vi "main.vi"() -> ()   [LabVIEW 2024]
uses:
  <vilib>/Utility/error.llb/DialogType.ctl
  <vilib>/DAQmx/read.llb/DAQmx Read (Analog 1D Wfm NChan NSamp).vi
  <vilib>/DAQmx/create/channels.llb/DAQmx Create Channel (AI-Voltage-Basic).vi
  <vilib>/DAQmx/configure/timing.llb/DAQmx Timing (Sample Clock).vi
  <vilib>/DAQmx/configure/task.llb/DAQmx Configure Logging (TDMS).vi
  <vilib>/DAQmx/configure/trigger.llb/DAQmx Start Trigger (Digital Edge).vi
  <vilib>/DAQmx/configure/trigger.llb/DAQmx Start Trigger (Time).vi
  <vilib>/DAQmx/configure/trigger.llb/DAQmx Start Trigger (Analog Edge).vi
  <vilib>/DAQmx/miscellaneous.llb/DAQmx Fill In Error Info.vi
  <vilib>/Utility/file.llb/Read Delimited Spreadsheet (string).vi
  <vilib>/Utility/file.llb/Write Delimited Spreadsheet (string).vi
  <vilib>/Utility/config.llb/Read Key (Double).vi
  <vilib>/Utility/config.llb/Read Key (I32).vi
  <vilib>/Utility/config.llb/Read Key (String).vi
  <vilib>/Utility/config.llb/Read Key (Path).vi
  <vilib>/Utility/config.llb/Write Key (Double).vi
  <vilib>/Utility/config.llb/Write Key (I32).vi
  <vilib>/Utility/config.llb/Write Key (String).vi
  <vilib>/Utility/config.llb/Write Key (Path).vi
  <resource>/objmgr/daqmx.rc
  <vilib>/Utility/config.llb/NI_LVConfig.lvlib
panel:
  in  "?":string(combo)
  out "Waveform Graph 2":waveform(dbl)[](graph)
  in  "?":string(combo)
  out "Waveform Graph":waveform(dbl)[](graph)
  out "子通道数":dbl[](array[numeric])
  in  "配置信息":enum32{"通道信息", "采样信息", "存储信息", "触发信息", "图表显示"}(tab)
  in  "通道信息":i32(listbox)
  in  "Sample Rate":dbl=1000.0
  out "Actual Sample Rate":dbl=1000.0 format="%0.2f"
  in  "Number of Samples":i32=100
  in  "Sample Clock Source":tag="OnboardClock"
  in  "Logging Mode":i32(ring)=10231 items=["Off"=10231, "Log and Read"=15842]
  in  "TDMS File Path":path
  in  "Trigger Type":T1(tab)
  in  "Digital Start Trigger Edge":i32(ring)=10280 caption="Edge" items=["Rising"=10280, "Falling"=10171]
  in  "Digital Start Trigger Source":tag="/Dev1/PFI0" caption="Source"
  in  "Digital Pause Trigger Pause When":i32(ring)=10192 caption="Pause When" items=["High"=10192, "Low"=10214]
  in  "Digital Pause Trigger Source":tag="/Dev1/PFI0" caption="Source"
  in  "Analog Start Trigger Level":dbl caption="Level" format="%0.2f"
  in  "Analog Start Trigger Hysteresis":dbl caption="Hysteresis" format="%.2f"
  in  "Analog Start Trigger Slope":i32(ring)=10280 caption="Slope" items=["Rising"=10280, "Falling"=10171]
  in  "Analog Start Trigger Source":string="APFI0" caption="Source"
  in  "Analog Pause Trigger Source":string="APFI0" caption="Source"
  in  "Analog Pause Trigger Pause When":i32(ring)=10093 caption="Pause When" items=["Above Level"=10093, "Below Level"=10107]
  in  "Analog Pause Trigger Level":dbl caption="Level" format="%.2f"
  in  "When":timestamp
  in  "Select Time\nManually":bool
  in  "横轴（显示时长）":dbl=1000.0
  out "采集状态":bool
  in  "开始采集":bool
  in  "Cluster":T2={"Terminal Configuration"=-1, "Min Voltage"=-5.0, "Physical Channel"="Dev1/ai0", "Max Voltage"=5.0, "function"="", "on/off"=FALSE, "物理量"="", "单位"=""} {"Terminal Configuration" items=["default"=-1, "RSE"=10083, "NRSE"=10078, "Differential"=10106, "Pseudodifferential"=12529]}
  out "Whole Waveform Graph":waveform(dbl)[](graph)
  in  "?":T3(array[cluster]) {"Terminal Configuration" items=["default"=-1, "RSE"=10083, "NRSE"=10078, "Differential"=10106, "Pseudodifferential"=12529]}
  # "All Channels"
  # "Timing Settings"
  # "Logging Settings"
  # "To enable triggers, select a tab above, and configure the settings.\n\nNot all hardware supports all trigger types. Refer to your device documentation for more information."
  # "This trigger type is not supported in continuous sample timing. \n\nRefer to your device documentation for more information on which triggers are supported."
  # "This trigger type is not supported in continuous sample timing. \n\nRefer to your device documentation for more information on which triggers are supported."
  # "If time is not manually set, task will begin after 10 seconds"
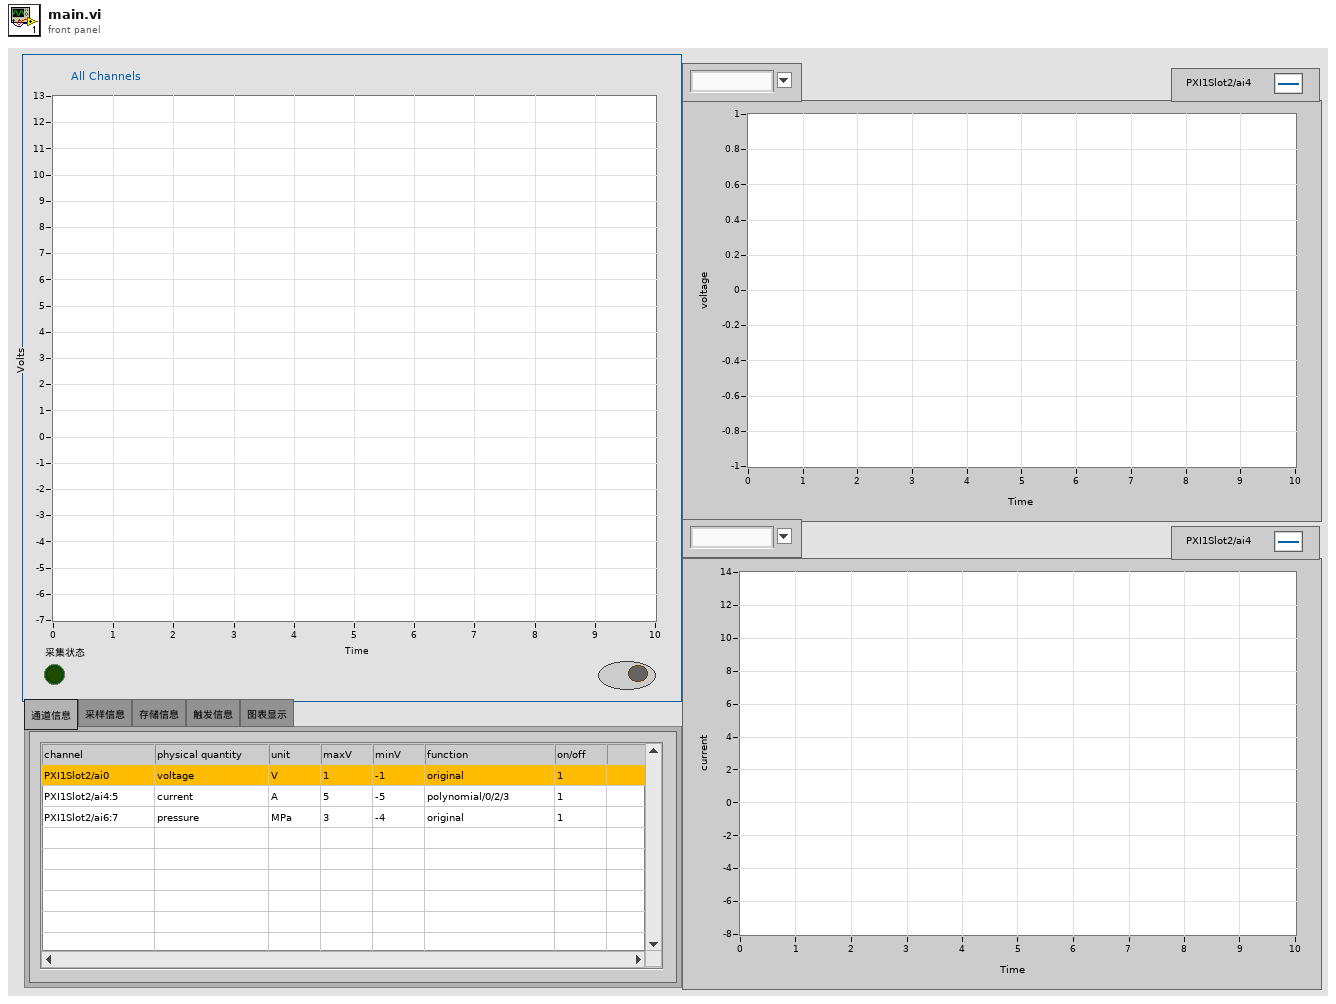
[diagram p1: front panel]
types:
  T1 = enum32{"No Trigger", "Digital Start", "Digital Pause", "Digital Reference", "Analog Start", "Analog Pause", "Analog Reference", "Time Start"}
  T2 = cluster{"Terminal Configuration":i32, "Min Voltage":dbl, "Physical Channel":tag, "Max Voltage":dbl, "function":string, "on/off":bool, "物理量":string, "单位":string}
  T3 = cluster{"Terminal Configuration":i32, "Min Voltage":dbl, "Physical Channel":tag, "Max Voltage":dbl, "function":string, "on/off":bool, "物理量":string, "单位":string}[]
  T4 = typedef "NI_LVConfig.lvlib/Config Data RefNum.ctl" = refnum<k1>
  T5 = typedef "DialogType.ctl" = u16
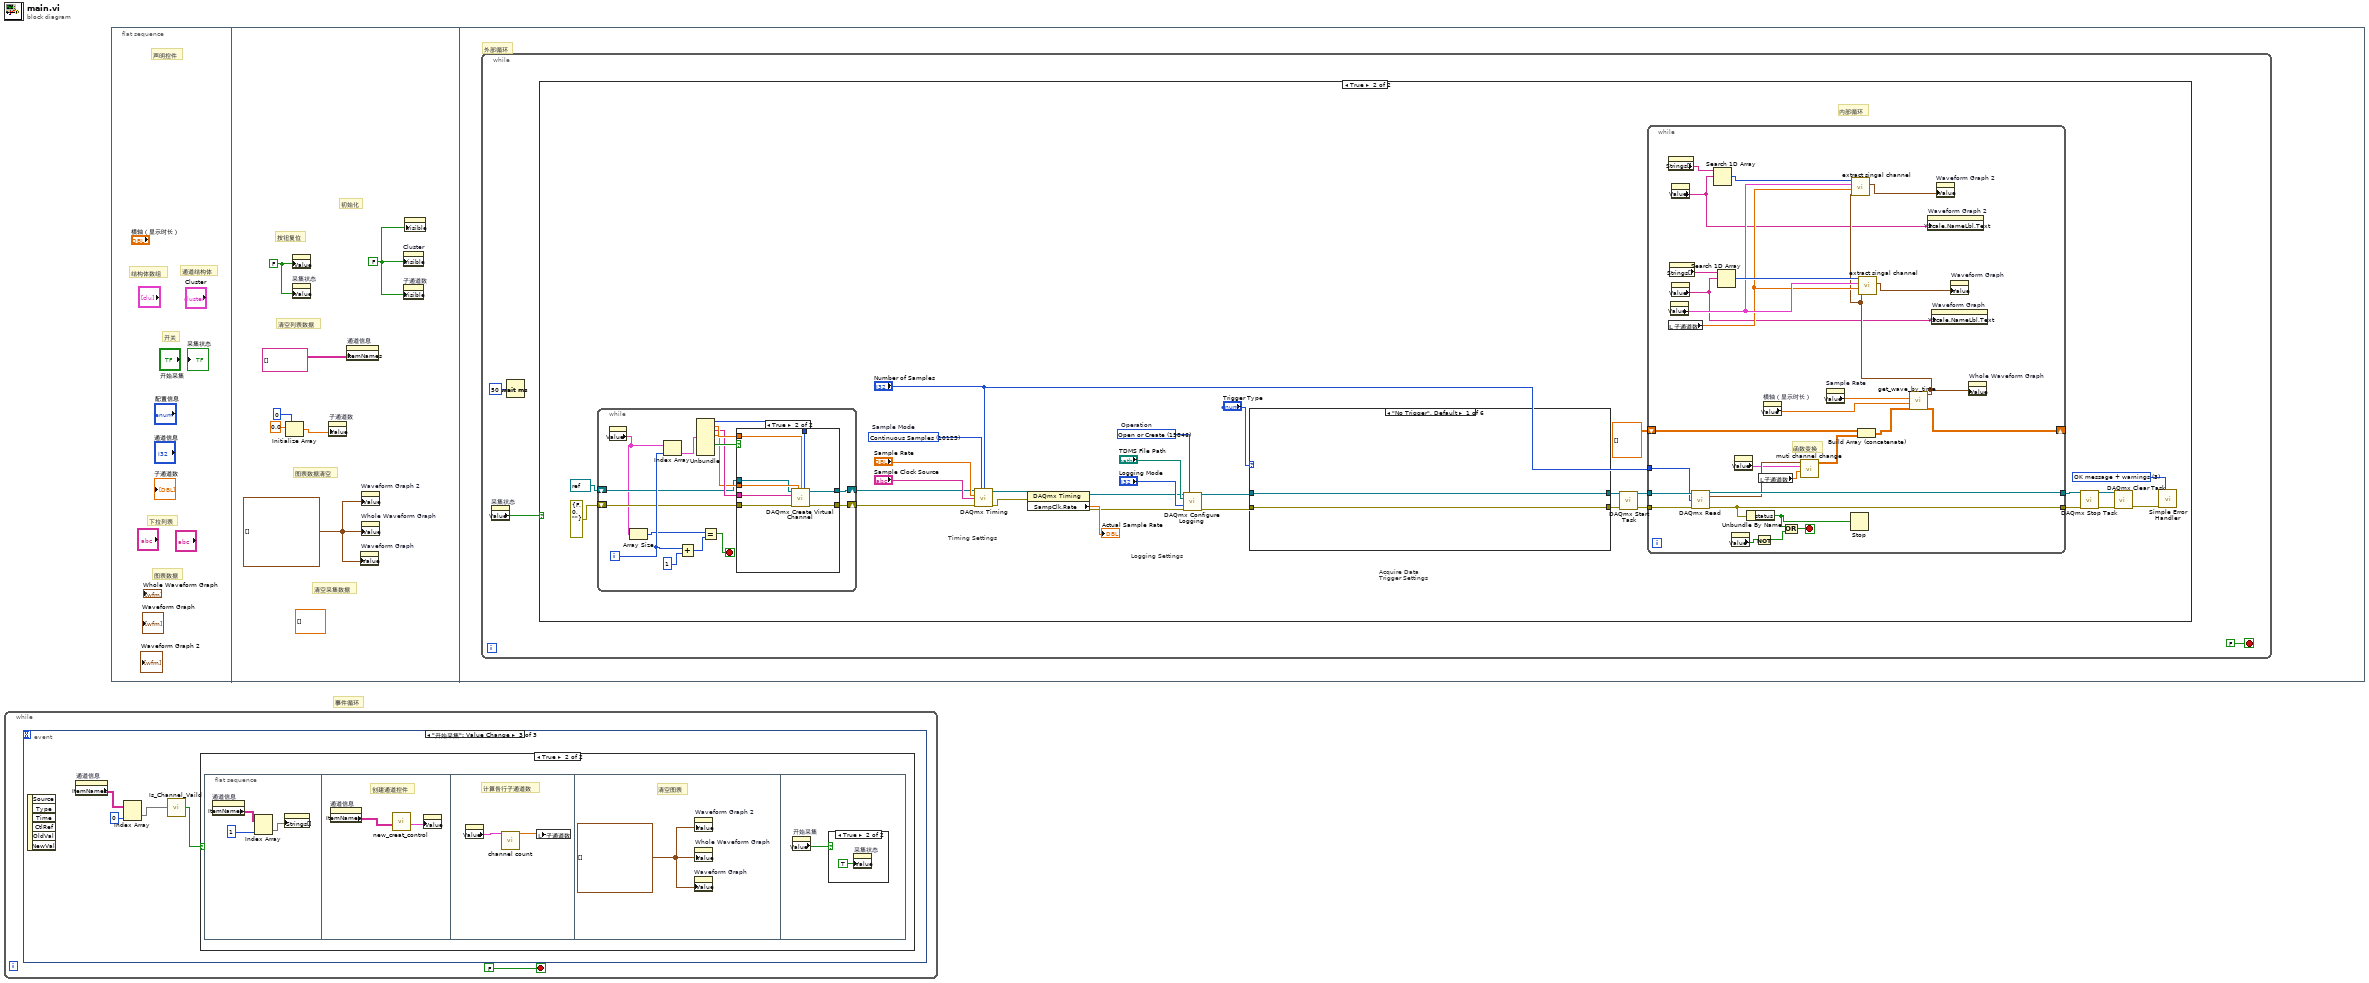
[diagram p0: block diagram]
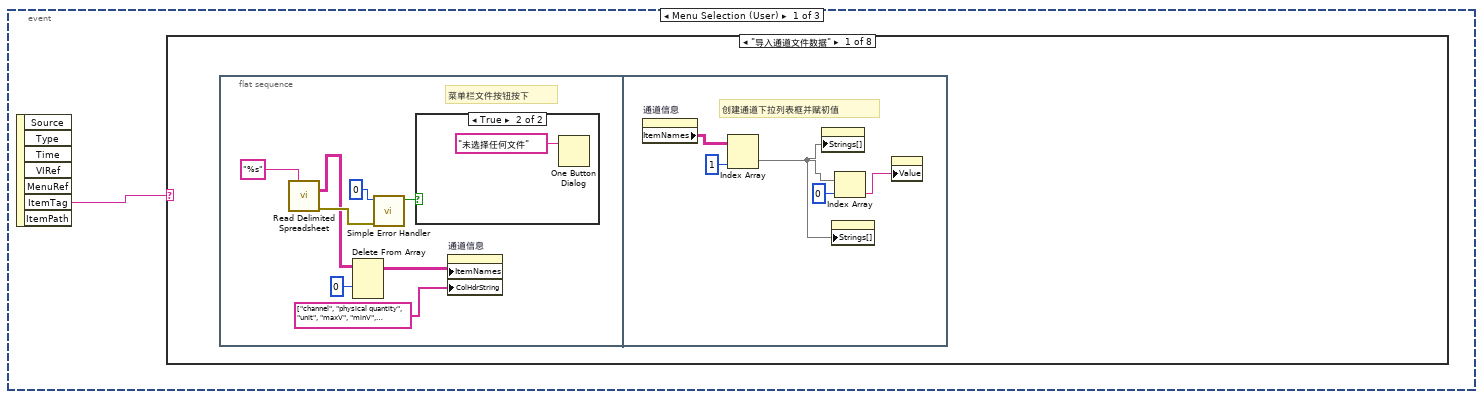
[diagram p2: hidden frame]
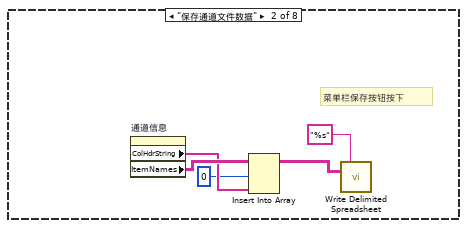
[diagram p4: hidden frame]
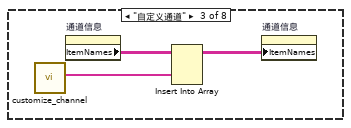
[diagram p5: hidden frame]
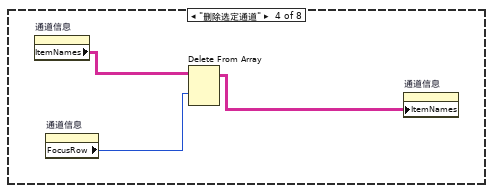
[diagram p6: hidden frame]
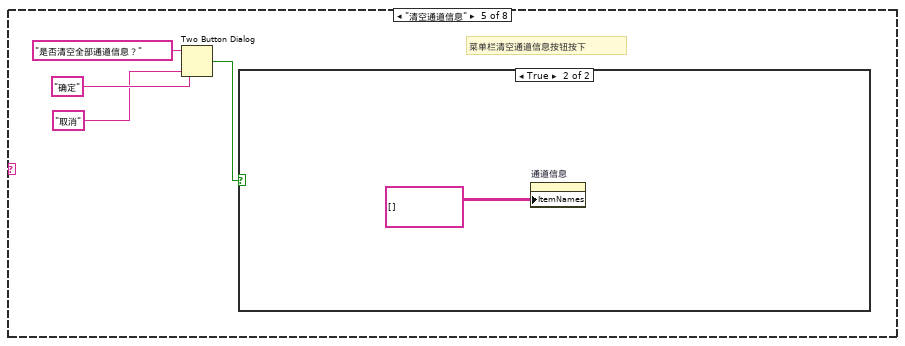
[diagram p7: hidden frame]
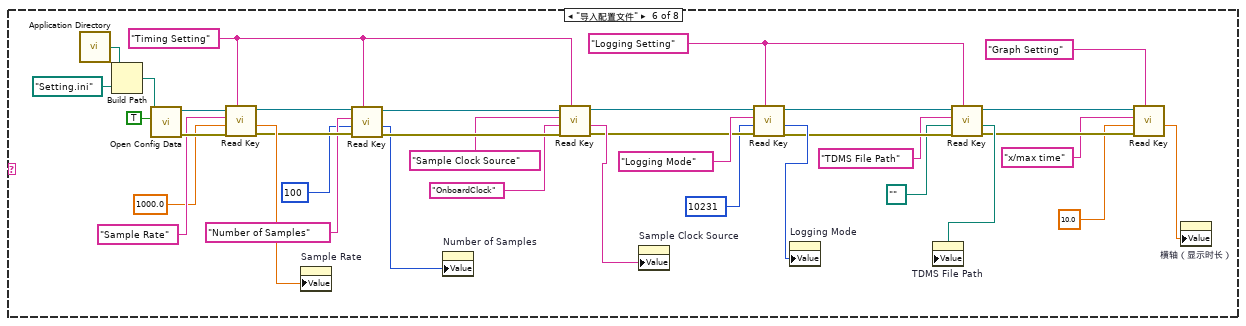
[diagram p9: hidden frame]
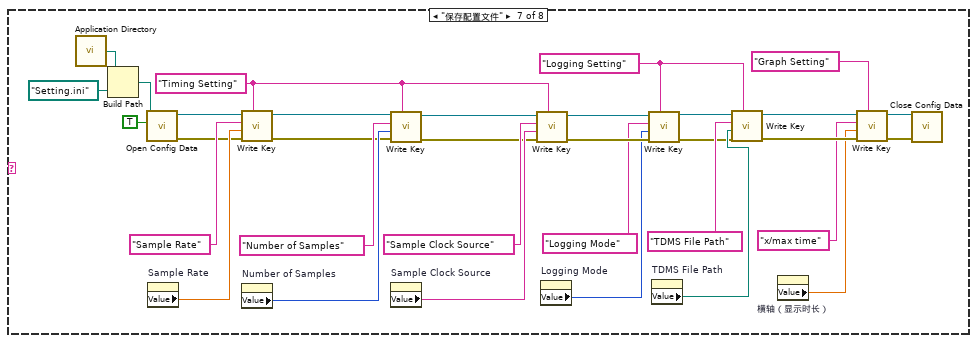
[diagram p10: hidden frame]
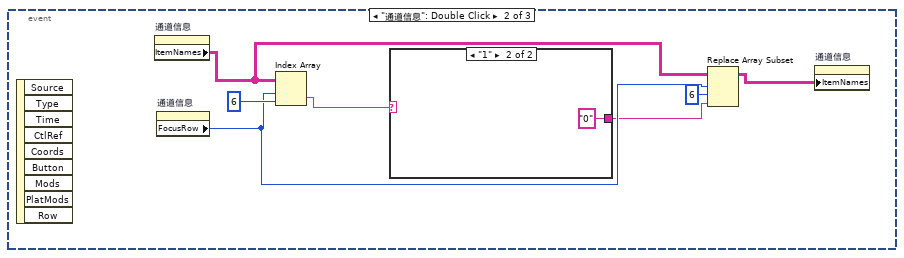
[diagram p12: hidden frame]
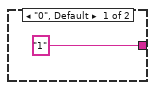
[diagram p13: hidden frame]
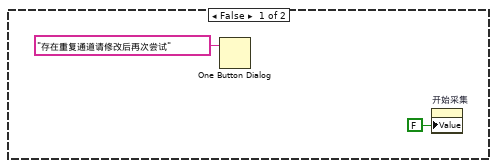
[diagram p14: hidden frame]
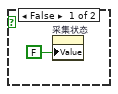
[diagram p15: hidden frame]
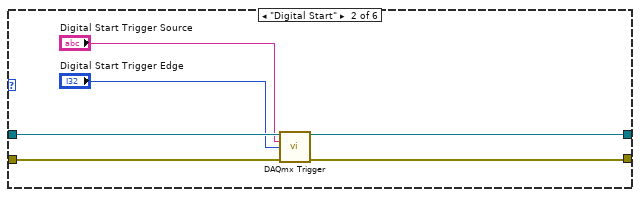
[diagram p17: hidden frame]
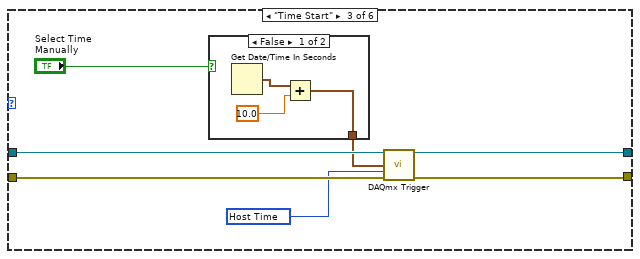
[diagram p18: hidden frame]
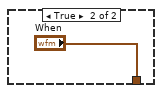
[diagram p19: hidden frame]
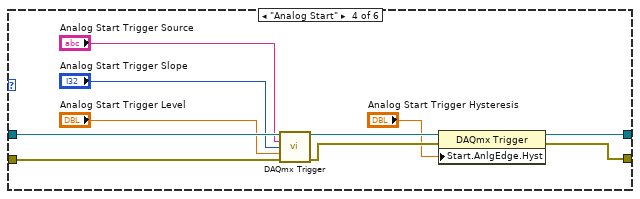
[diagram p20: hidden frame]
diagram:
  # "事件循环"
  n1 = while {
    stop <- FALSE stop-if-true
    n2 = event shown="[2] \"开始采集\": Value Change" {
      selector: _ -> [_ _ _]
      dyn-events: _ -> [_ _ _]
      timeout: _ -> [_ _ _]
      event Menu Selection (User) {
        n3 = event-data() -> ("ItemTag"=w2:string)  [unwired: 1 in, 6 out]
        n4 = case shown="\"导入通道文件数据\"" w2 {
          frame "导入通道文件数据" {
            n5 = flat-sequence {
              frame #0 {
                # "菜单栏文件按钮按下"
                n6 = call-poly <vilib>:"Read Delimited Spreadsheet.vi"("format (%s)"="%s") -> ("all rows"=w8:string[][], "error out"=w10:errorcluster)  [unwired: 9 in, 4 out]
                n7 = Delete From Array(array=w8, index (row)=0) -> (array with subset deleted=w7:string[][])  [unwired: 2 in, 1 out]
                n8 = call <vilib>:"Simple Error Handler.vi"("error code (no error:0)"=0, "error in (no error)"=w10) -> ("error?"=w9:bool)  [unwired: 3 in, 4 out]
                n9 = case shown="True" w9 {
                  frame False {
                  }
                  frame True {
                    n10 = One Button Dialog(message="未选择任何文件") -> ()  [unwired: 1 in, 1 out]
                  }
                }
                n11 = property on="通道信息" class="MCListbox (strict)"("ItemNames"=w7, "ColHdrString"=string[] ["channel", "physical quantity", "unit", "maxV", "minV", "function", "on/off"]) -> ()  [unwired: 2 in, 2 out]
              }
              frame #1 {
                # "创建通道下拉列表框并赋初值"
                n12 = property on="通道信息" class="MCListbox (strict)"() -> ("ItemNames"=w16:string[][])  [unwired: 2 in, 2 out]
                n13 = Index Array(array=w16, index (col)=1 ("disabled index (col)")) -> (element=w12:string[])  [unwired: 1 in]
                n14 = property class="CmbBox"("Strings[]"=w12) -> ()  [unwired: 2 in, 2 out]
                n15 = property class="CmbBox"("Strings[]"=w12) -> ()  [unwired: 2 in, 2 out]
                n16 = Index Array(array=w12, index=0) -> (element=w13:string)
                n17 = property class="CmbBox"("Value"=w13) -> ()  [unwired: 2 in, 2 out]
              }
            }
          }
          frame "保存通道文件数据" {
            # "菜单栏保存按钮按下"
            n18 = property on="通道信息" class="MCListbox (strict)"() -> ("ColHdrString"=w19:string[], "ItemNames"=w20:string[][])  [unwired: 2 in, 2 out]
            n19 = Insert Into Array(array=w20, index (row)=0, new element=w19) -> (w17:string[][])  [unwired: 1 in]
            n20 = call-poly <vilib>:"Write Delimited Spreadsheet.vi"("format (%s)"="%s", "2D data"=w17) -> ()  [unwired: 12 in, 2 out]
          }
          frame "自定义通道" {
            n21 = call "customize_channel.vi"() -> ("Array - String"=w24:string[])  [unwired: 11 in]
            n22 = property on="通道信息" class="MCListbox (strict)"() -> ("ItemNames"=w23:string[][])  [unwired: 2 in, 2 out]
            n23 = Insert Into Array(array=w23, new element=w24) -> (w22:string[][])  [unwired: 2 in]
            n24 = property on="通道信息" class="MCListbox (strict)"("ItemNames"=w22) -> ()  [unwired: 2 in, 2 out]
          }
          frame "删除选定通道" {
            n25 = property on="通道信息" class="MCListbox (strict)"() -> ("ItemNames"=w27:string[][])  [unwired: 2 in, 2 out]
            n26 = property on="通道信息" class="MCListbox (strict)"() -> ("FocusRow"=w26:i32)  [unwired: 2 in, 2 out]
            n27 = Delete From Array(array=w27, index (row)=w26) -> (array with subset deleted=w25:string[][])  [unwired: 2 in, 1 out]
            n28 = property on="通道信息" class="MCListbox (strict)"("ItemNames"=w25) -> ()  [unwired: 2 in, 2 out]
          }
          frame "清空通道信息" {
            # "菜单栏清空通道信息按钮按下"
            n29 = Two Button Dialog(message="是否清空全部通道信息？", 1:"取消" ("F button name (\"Cancel\")"), 2:"确定" ("T button name (\"OK\")")) -> (T button?=w28:bool)
            n30 = case shown="True" w28 {
              frame False {
              }
              frame True {
                n31 = property on="通道信息" class="MCListbox (strict)"("ItemNames"=string[][] []) -> ()  [unwired: 2 in, 2 out]
              }
            }
          }
          frame "导入配置文件" {
            w41 = "Logging Setting" ("section")
            w54 = "Timing Setting" ("section")
            n32 = call <vilib>:"Application Directory.vi"() -> ("Application Directory"=w69:path)
            n33 = Build Path(base path=w69, name or relative path=path "Setting.ini") -> (appended path=w68:path)
            n34 = call <vilib>:"Open Config Data.vi"("create file if necessary (T)"=TRUE, "configuration file path"=w68) -> ("error out"=w64:errorcluster, "refnum"=w65:T4)  [unwired: 7 in, 1 out]
            n35 = call-poly <vilib>:"Read Key.vi"("section"=w54, "error in (no error)"=w64, "default value"=1000.0, "key"="Sample Rate", "refnum"=w65) -> ("error out"=w60:errorcluster, "value"=w62:dbl, "refnum out"=w61:T4)  [unwired: 3 in, 1 out]
            n36 = property on="Sample Rate" class="DigNum (strict)"("Value"=w62) -> ()  [unwired: 2 in, 2 out]
            n37 = call-poly <vilib>:"Read Key.vi"("section"=w54, "error in (no error)"=w60, "default value"=100, "key"="Number of Samples", "refnum"=w61) -> ("error out"=w55:errorcluster, "value"=w53:i32, "refnum out"=w56:T4)  [unwired: 3 in, 1 out]
            n38 = property on="Number of Samples" class="DigNum (strict)"("Value"=w53) -> ()  [unwired: 2 in, 2 out]
            n39 = call-poly <vilib>:"Read Key.vi"("section"=w54, "error in (no error)"=w55, "default value"="OnboardClock", "key"="Sample Clock Source", "refnum"=w56) -> ("error out"=w47:errorcluster, "value"=w50:string, "refnum out"=w48:T4)  [unwired: 3 in, 1 out]
            n40 = property on="Sample Clock Source" class="DAQmxName"("Value"=w50) -> ()  [unwired: 2 in, 2 out]
            n41 = call-poly <vilib>:"Read Key.vi"("section"=w41, "error in (no error)"=w47, "default value"=10231, "key"="Logging Mode", "refnum"=w48) -> ("error out"=w43:errorcluster, "value"=w46:i32, "refnum out"=w44:T4)  [unwired: 3 in, 1 out]
            n42 = property on="Logging Mode" class="Ring (strict)"("Value"=w46) -> ()  [unwired: 2 in, 2 out]
            n43 = call-poly <vilib>:"Read Key.vi"("section"=w41, "error in (no error)"=w43, "default value"=path "", "key"="TDMS File Path", "refnum"=w44) -> ("error out"=w37:errorcluster, "value"=w40:path, "refnum out"=w38:T4)  [unwired: 3 in, 1 out]
            n44 = property on="TDMS File Path" class="Path"("Value"=w40) -> ()  [unwired: 2 in, 2 out]
            n45 = call-poly <vilib>:"Read Key.vi"("section"="Graph Setting", "error in (no error)"=w37, "default value"=10.0, "key"="x/max time", "refnum"=w38) -> ("value"=w34:dbl)  [unwired: 3 in, 3 out]
            n46 = property on="横轴（显示时长）" class="DigNum (strict)"("Value"=w34) -> ()  [unwired: 2 in, 2 out]
          }
          frame "保存配置文件" {
            w81 = "Logging Setting" ("section")
            w92 = "Timing Setting" ("section")
            n47 = call <vilib>:"Application Directory.vi"() -> ("Application Directory"=w88:path)
            n48 = Build Path(base path=w88, name or relative path=path "Setting.ini") -> (appended path=w86:path)
            n49 = call <vilib>:"Open Config Data.vi"("create file if necessary (T)"=TRUE, "configuration file path"=w86) -> ("error out"=w91:errorcluster, "refnum"=w101:T4)  [unwired: 7 in, 1 out]
            n50 = property on="Sample Rate" class="DigNum (strict)"() -> ("Value"=w99:dbl)  [unwired: 2 in, 2 out]
            n51 = call-poly <vilib>:"Write Key.vi"("section"=w92, "error in (no error)"=w91, "value"=w99, "key"="Sample Rate", "refnum"=w101) -> ("error out"=w90:errorcluster, "refnum out"=w98:T4)  [unwired: 4 in, 1 out]
            n52 = property on="Number of Samples" class="DigNum (strict)"() -> ("Value"=w97:i32)  [unwired: 2 in, 2 out]
            n53 = call-poly <vilib>:"Write Key.vi"("section"=w92, "error in (no error)"=w90, "value"=w97, "key"="Number of Samples", "refnum"=w98) -> ("error out"=w89:errorcluster, "refnum out"=w93:T4)  [unwired: 4 in, 1 out]
            n54 = property on="Sample Clock Source" class="DAQmxName"() -> ("Value"=w95:string)  [unwired: 2 in, 2 out]
            n55 = call-poly <vilib>:"Write Key.vi"("section"=w92, "error in (no error)"=w89, "value"=w95, "key"="Sample Clock Source", "refnum"=w93) -> ("error out"=w84:errorcluster, "refnum out"=w85:T4)  [unwired: 4 in, 1 out]
            n56 = property on="Logging Mode" class="Ring (strict)"() -> ("Value"=w83:i32)  [unwired: 2 in, 2 out]
            n57 = call-poly <vilib>:"Write Key.vi"("section"=w81, "error in (no error)"=w84, "value"=w83, "key"="Logging Mode", "refnum"=w85) -> ("error out"=w77:errorcluster, "refnum out"=w78:T4)  [unwired: 4 in, 1 out]
            n58 = property on="TDMS File Path" class="Path"() -> ("Value"=w79:path)  [unwired: 2 in, 2 out]
            n59 = call-poly <vilib>:"Write Key.vi"("section"=w81, "error in (no error)"=w77, "value"=w79, "key"="TDMS File Path", "refnum"=w78) -> ("error out"=w75:errorcluster, "refnum out"=w76:T4)  [unwired: 4 in, 1 out]
            n60 = property on="横轴（显示时长）" class="DigNum (strict)"() -> ("Value"=w73:dbl)  [unwired: 2 in, 2 out]
            n61 = call-poly <vilib>:"Write Key.vi"("section"="Graph Setting", "error in (no error)"=w75, "value"=w73, "key"="x/max time", "refnum"=w76) -> ("error out"=w70:errorcluster, "refnum out"=w71:T4)  [unwired: 4 in, 1 out]
            n62 = call <vilib>:"Close Config Data.vi"("error in (no error)"=w70, "refnum"=w71) -> ()  [unwired: 8 in, 2 out]
          }
          frame "False", Default {
          }
        }
      }
      event "通道信息": Double Click {
        n63 = event-data() -> ()  [unwired: 1 in, 9 out]
        n64 = property on="通道信息" class="MCListbox (strict)"() -> ("ItemNames"=w107:string[][])  [unwired: 2 in, 2 out]
        n65 = property on="通道信息" class="MCListbox (strict)"() -> ("FocusRow"=w105:i32)  [unwired: 2 in, 2 out]
        n66 = Index Array(array=w107, index (row)=w105, index (col)=6 ("disabled index (col)")) -> (element=w108:string)
        n67 = case shown="\"1\"" w108 {
          tunnel: ["1" ("new element/subarray") "0" ("new element/subarray")] -> w104
          frame "0", Default {
          }
          frame "1" {
          }
        }
        n68 = Replace Array Subset(array=w107, new element=w104, index (row)=w105, index (col)=6 ("disabled index (col)")) -> (w103:string[][])
        n69 = property on="通道信息" class="MCListbox (strict)"("ItemNames"=w103) -> ()  [unwired: 2 in, 2 out]
      }
      event "开始采集": Value Change {
        n70 = event-data() -> ()  [unwired: 1 in, 6 out]
        n71 = property on="通道信息" class="MCListbox (strict)"() -> ("ItemNames"=w114:string[][])  [unwired: 2 in, 2 out]
        n72 = Index Array(array=w114, index (col)=0 ("disabled index (col)")) -> (element=w115:string[])  [unwired: 1 in]
        n73 = call "Is_Channel_Vaild.vi"("输入数组"=w115) -> ("元素不重复？（真：不重复，假：有重复元素）"=w112:bool)
        n74 = case shown="True" w112 {
          frame False {
            n75 = One Button Dialog(message="存在重复通道请修改后再次尝试") -> ()  [unwired: 1 in, 1 out]
            n76 = property on="开始采集" class="Bool (strict)"("Value"=FALSE ("开始采集")) -> ()  [unwired: 2 in, 2 out]
          }
          frame True {
            n77 = flat-sequence {
              frame #0 {
                n78 = property on="通道信息" class="MCListbox (strict)"() -> ("ItemNames"=w119:string[][])  [unwired: 2 in, 2 out]
                n79 = Index Array(array=w119, index (col)=1) -> (element=w118:string[])  [unwired: 1 in]
                n80 = property class="CmbBox"("Strings[]"=w118) -> ()  [unwired: 2 in, 2 out]
              }
              frame #1 {
                # "创建通道控件"
                n81 = property on="通道信息" class="MCListbox (strict)"() -> ("ItemNames"=w121:string[][])  [unwired: 2 in, 2 out]
                n82 = call "new_creat_control.vi"("Table"=w121) -> ("Array"=w122:T3)  [unwired: 10 in]
                n83 = property class="Arr (strict)"("Value"=w122) -> ()  [unwired: 2 in, 2 out]
              }
              frame #2 {
                # "计算各行子通道数"
                n84 = property class="Arr (strict)"() -> ("Value"=w124:T3)  [unwired: 2 in, 2 out]
                n85 = call "channel count.vi"(11:w124) -> ("Array - Numeric"=w123:dbl[])  [unwired: 10 in]
                n86 = local write "子通道数"(w123) -> ()
              }
              frame #3 {
                w125 = waveform(dbl)[] [] ("Whole Waveform Graph")
                # "清空图表"
                n87 = property on="Waveform Graph" class="WFGraph (strict)"("Value"=w125) -> ()  [unwired: 2 in, 2 out]
                n88 = property on="Waveform Graph 2" class="WFGraph (strict)"("Value"=w125) -> ()  [unwired: 2 in, 2 out]
                n89 = property on="Whole Waveform Graph" class="WFGraph (strict)"("Value"=w125) -> ()  [unwired: 2 in, 2 out]
              }
              frame #4 {
                n90 = property on="开始采集" class="Bool (strict)"() -> ("Value"=w126:bool)  [unwired: 2 in, 2 out]
                n91 = case shown="True" w126 {
                  frame False {
                    n92 = property on="采集状态" class="Bool (strict)"("Value"=FALSE) -> ()  [unwired: 2 in, 2 out]
                  }
                  frame True {
                    n93 = property on="采集状态" class="Bool (strict)"("Value"=TRUE) -> ()  [unwired: 2 in, 2 out]
                  }
                }
              }
            }
          }
        }
      }
    }
  }
  n94 = flat-sequence {
    frame #0 {
      # "图表数据"
      # "下拉列表"
      # "声明控件"
      # "开关"
      # "结构体数组"
      # "通道结构体"
    }
    frame #1 {
      (unwired) dbl[][] [] ("statistic")
      w129 = waveform(dbl)[] [] ("Whole Waveform Graph")
      w130 = FALSE
      w135 = FALSE ("on/off")
      # "清空采集数据"
      # "图表数据清空"
      # "清空列表数据"
      # "初始化"
      # "按钮复位"
      n95 = Initialize Array(0.0 ("element"), 0 ("dimension size")) -> (w133:dbl[])
      n96 = property on="开始采集" class="Bool (strict)"("Value"=w135) -> ()  [unwired: 2 in, 2 out]
      n97 = property on="采集状态" class="Bool (strict)"("Value"=w135) -> ()  [unwired: 2 in, 2 out]
      n98 = property on="子通道数" class="Arr (strict)"("Value"=w133) -> ()  [unwired: 2 in, 2 out]
      n99 = property on="通道信息" class="MCListbox (strict)"("ItemNames"=string[][] []) -> ()  [unwired: 2 in, 2 out]
      n100 = property on="Waveform Graph" class="WFGraph (strict)"("Value"=w129) -> ()  [unwired: 2 in, 2 out]
      n101 = property on="Waveform Graph 2" class="WFGraph (strict)"("Value"=w129) -> ()  [unwired: 2 in, 2 out]
      n102 = property on="Whole Waveform Graph" class="WFGraph (strict)"("Value"=w129) -> ()  [unwired: 2 in, 2 out]
      n103 = property on="Cluster" class="Clust (strict)"("Visible"=w130) -> ()  [unwired: 2 in, 2 out]
      n104 = property on="子通道数" class="Arr (strict)"("Visible"=w130) -> ()  [unwired: 2 in, 2 out]
      n105 = property class="Arr (strict)"("Visible"=w130) -> ()  [unwired: 2 in, 2 out]
    }
    frame #2 {
      # "外部循环"
      n106 = while {
        stop <- FALSE stop-if-true
        n107 = property on="采集状态" class="Bool (strict)"() -> ("Value"=w136:bool)  [unwired: 2 in, 2 out]
        n108 = Wait (ms)(milliseconds to wait=u32 50) -> ()  [unwired: 1 out]
        n109 = case shown="True" w136 {
          frame False {
          }
          frame True {
            w161 = T5 3 items=["no dialog", "OK message", "continue or stop message", "OK message + warnings", "continue/stop + warnings"] ("type of dialog (OK msg:1)")
            w147 = 15846 items=["Open"=10437, "Open or Create"=15846, "Create or Replace"=15847, "Create"=15848]  # Operation
            w144 = 10123 items=["Finite Samples"=10178, "Continuous Samples"=10123, "Hardware Timed Single Point"=12522]  # Sample Mode
            # "内部循环"
            # "Trigger Settings"
            # "Acquire Data"
            # "Timing Settings"
            # "Logging Settings"
            n110 = while {
              shift-right: [w246] -> w141
              shift-left: refnum<k21> refnum ("task out") -> [w243]
              shift-right: [w245] -> w140
              shift-left: errorcluster {"status"=FALSE, "code"=0, "source"=""} ("error out") -> [w244]
              i -> [w257]
              stop <- w254 stop-if-true
              n111 = property class="Arr (strict)"() -> ("Value"=w242:T3)  [unwired: 2 in, 2 out]
              n112 = Array Size(array=w242) -> (size(s)=w251:i32)
              n113 = Index Array(array=w242, index=w257) -> (element=w253:T2)
              n114 = Add(x=w257, y=1) -> (x+y=w255:i32)
              n115 = Unbundle(w253) -> ("Terminal Configuration"=w250:i32, "Min Voltage"=w249:dbl, "Physical Channel"=w248:tag, "Max Voltage"=w247:dbl, "on/off"=w252:bool)  [unwired: 3 out]
              n116 = Equal?(x=w251, y=w255) -> (x = y?=w254:bool)
              n117 = case shown="True" w252 {
                tunnel: w250 -> [_ w267]
                tunnel: w249 -> [_ w266]
                tunnel: w248 -> [_ w265]
                tunnel: w247 -> [_ w264]
                tunnel: [w259 w263] -> w246
                tunnel: [w258 w262] -> w245
                tunnel: w244 -> [w258 w261]
                tunnel: w243 -> [w259 w260]
                frame False {
                }
                frame True {
                  n118 = call-poly <vilib>:"DAQmx Create Virtual Channel.vi"("task in"=w260, "maximum value"=w264, "minimum value"=w266, "input terminal configuration"=w267, "physical channels"=w265, "error in"=w261) -> ("task out"=w263:refnum<k21>, "error out"=w262:errorcluster)  [unwired: 8 in]
                }
              }
            }
            n119 = call-poly <vilib>:"DAQmx Timing.vi"("task/channels in"=w141, "sample mode"=w144, "samples per channel"="Number of Samples", "rate"="Sample Rate", "source"="Sample Clock Source", "error in"=w140) -> ("task out"=w142:refnum<k21>, "error out"=w143:errorcluster)  [unwired: 8 in]
            n120 = property class="DAQmx Timing"(reference=w142, error in=w143) -> (reference out=w145:refnum<k21>, error out=w146:errorcluster, "SampClk.Rate"=→"Actual Sample Rate":dbl)
            n121 = call-poly <vilib>:"DAQmx Configure Logging.vi"("task/channels in"=w145, "operation"=w147, "file path"="TDMS File Path", "logging mode"="Logging Mode", "error in"=w146) -> ("task out"=w163:refnum<k21>, "error out"=w164:errorcluster)  [unwired: 9 in]
            n122 = case shown="\"No Trigger\", Default" "Trigger Type" {
              tunnel: w163 -> [w170 w176 w183 w197 w204 w212]
              tunnel: w164 -> [w169 w175 w182 w196 w201 w209]
              tunnel: [w170 w174 w181 w194 w203 w211] -> w166
              tunnel: [w169 w173 w180 w193 w202 w210] -> w165
              frame "No Trigger", Default {
              }
              frame "Digital Start" {
                n123 = call-poly <vilib>:"DAQmx Trigger.vi"("task/channels in"=w176, "source"="Digital Start Trigger Source", "edge"="Digital Start Trigger Edge", "error in"=w175) -> ("task out"=w174:refnum<k21>, "error out"=w173:errorcluster)  [unwired: 10 in]
              }
              frame "Time Start" {
                w179 = 16126 items=["Host Time"=16126, "I/O Device Time"=16127] ("timescale")
                n124 = case shown="False" "Select Time\nManually" {
                  tunnel: [w184 "When"] -> w177
                  frame False {
                    n125 = Get Date/Time In Seconds() -> (seconds since 1Jan1904=w186:timestamp)
                    n126 = Add(x=w186, y=10.0) -> (x+y=w184:timestamp)
                  }
                  frame True {
                  }
                }
                n127 = call-poly <vilib>:"DAQmx Trigger.vi"("task/channels in"=w183, "when"=w177, "timescale"=w179, "error in"=w182) -> ("task out"=w181:refnum<k21>, "error out"=w180:errorcluster)  [unwired: 10 in]
              }
              frame "Analog Start" {
                n128 = call-poly <vilib>:"DAQmx Trigger.vi"("task/channels in"=w197, "source"="Analog Start Trigger Source", "slope"="Analog Start Trigger Slope", "level"="Analog Start Trigger Level", "error in"=w196) -> ("task out"=w192:refnum<k21>, "error out"=w191:errorcluster)  [unwired: 9 in]
                n129 = property class="DAQmx Trigger"(reference=w192, error in=w191, "Start.AnlgEdge.Hyst"="Analog Start Trigger Hysteresis") -> (reference out=w194:refnum<k21>, error out=w193:errorcluster)
              }
              frame "Digital Pause" {
                w200 = 10152 items=["Analog Level"=10101, "Analog Window"=10103, "Digital Level"=10152, "Digital Pattern"=10398, "None"=10230] ("Pause.TrigType")
                n130 = property class="DAQmx Trigger"(reference=w204, error in=w201, "Pause.TrigType"=w200, "More:Pause:Digital Level:Source"="Digital Pause Trigger Source", "More:Pause:Digital Level:Pause When"="Digital Pause Trigger Pause When") -> (reference out=w203:refnum<k21>, error out=w202:errorcluster)
              }
              frame "Analog Pause" {
                w208 = 10101 items=["Analog Level"=10101, "Analog Window"=10103, "Digital Level"=10152, "Digital Pattern"=10398, "None"=10230] ("Pause.TrigType")
                n131 = property class="DAQmx Trigger"(reference=w212, error in=w209, "Pause.TrigType"=w208, "Pause.AnlgLvl.Src"="Analog Pause Trigger Source", "Pause.AnlgLvl.When"="Analog Pause Trigger Pause When", "Pause.AnlgLvl.Lvl"="Analog Pause Trigger Level") -> (reference out=w211:refnum<k21>, error out=w210:errorcluster)
              }
            }
            n132 = call <vilib>:"DAQmx Start Task.vi"("task/channels in"=w166, "error in"=w165) -> ("task out"=w148:refnum<k21>, "error out"=w149:errorcluster)  [unwired: 12 in]
            n133 = while {
              tunnel: w148 -> [w241]
              tunnel: w149 -> [w240]
              tunnel: [w239] -> w157
              tunnel: [w238] -> w158
              tunnel: "Number of Samples" -> [w236]
              shift-right: [w222] -> _
              shift-left: dbl[][][] [] ("new array") -> [w226]
              stop <- w237 stop-if-true
              # "函数变换"
              n134 = property class="CmbBox"() -> ("Strings[]"=w220:string[])  [unwired: 2 in, 2 out]
              n135 = local read "子通道数"() -> (w217:dbl[])
              n136 = property class="CmbBox"() -> ("Strings[]"=w232:string[])  [unwired: 2 in, 2 out]
              n137 = property class="Arr (strict)"() -> ("Value"=w218:T3)  [unwired: 2 in, 2 out]
              n138 = property class="CmbBox"() -> ("Value"=w213:string)  [unwired: 2 in, 2 out]
              n139 = property class="CmbBox"() -> ("Value"=w214:string)  [unwired: 2 in, 2 out]
              n140 = call-poly <vilib>:"DAQmx Read.vi"("task/channels in"=w241, "number of samples per channel"=w236, "error in"=w240) -> ("task out"=w239:refnum<k21>, "data"=w230:waveform(dbl)[], "error out"=w238:errorcluster)  [unwired: 10 in]
              n141 = Search 1D Array(1D array=w220, element=w213) -> (index of element=w219:i32)  [unwired: 1 in]
              n142 = Search 1D Array(1D array=w232, element=w214) -> (index of element=w231:i32)  [unwired: 1 in]
              n143 = property on="开始采集" class="Bool (strict)"() -> ("Value"=w234:bool)  [unwired: 2 in, 2 out]
              n144 = property class="Arr (strict)"() -> ("Value"=w229:T3)  [unwired: 2 in, 2 out]
              n145 = Unbundle By Name(w238) -> ("status"=w235:bool)
              n146 = Not(x=w234) -> (.not. x?=w233:bool)
              n147 = local read "子通道数"() -> (w228:dbl[])
              n148 = property on="横轴（显示时长）" class="DigNum (strict)"() -> ("Value"=w224:dbl)  [unwired: 2 in, 2 out]
              n149 = Or(x=w235, y=w233) -> (x .or. y?=w237:bool)
              n150 = call "muti channel change.vi"("Array - Numeric"=w228, 9:w229, "data in"=w230) -> ("data out"=w227:dbl[][])  [unwired: 7 in]
              n151 = property on="Sample Rate" class="DigNum (strict)"() -> ("Value"=w223:dbl)  [unwired: 2 in, 2 out]
              n152 = Stop(stop? (T)=w235) -> ()
              n153 = Build Array (concatenate)(w226, w227) -> (w225:dbl[][][])
              n154 = call "get_wave_by_time.vi"("Sample Rate"=w223, "横轴（显示时长）"=w224, "appended array"=w225) -> ("data"=w216:waveform(dbl)[], "new array"=w222:dbl[][][])  [unwired: 5 in]
              n155 = call "extract singal channel.vi"("data in"=w216, "Array - Numeric"=w217, 10:w218, "channel index"=w219) -> ("data out"=w215:waveform(dbl)[])  [unwired: 7 in]
              n156 = call "extract singal channel.vi"("data in"=w216, "Array - Numeric"=w217, 10:w218, "channel index"=w231) -> ("data out"=w221:waveform(dbl)[])  [unwired: 7 in]
              n157 = property on="Waveform Graph 2" class="WFGraph (strict)"("YScale.NameLbl.Text"=w213) -> ()  [unwired: 2 in, 2 out]
              n158 = property on="Waveform Graph" class="WFGraph (strict)"("YScale.NameLbl.Text"=w214) -> ()  [unwired: 2 in, 2 out]
              n159 = property on="Waveform Graph 2" class="WFGraph (strict)"("Value"=w215) -> ()  [unwired: 2 in, 2 out]
              n160 = property on="Waveform Graph" class="WFGraph (strict)"("Value"=w221) -> ()  [unwired: 2 in, 2 out]
              n161 = property on="Whole Waveform Graph" class="WFGraph (strict)"("Value"=w216) -> ()  [unwired: 2 in, 2 out]
            }
            n162 = call <vilib>:"DAQmx Stop Task.vi"("task/channels in"=w157, "error in"=w158) -> ("task out"=w160:refnum<k21>, "error out"=w159:errorcluster)  [unwired: 12 in]
            n163 = call <vilib>:"DAQmx Clear Task.vi"("task in"=w160, "error in"=w159) -> ("error out"=w150:errorcluster)  [unwired: 13 in]
            n164 = call <vilib>:"Simple Error Handler.vi"("type of dialog (OK msg:1)"=w161, "error in (no error)"=w150) -> ()  [unwired: 3 in, 5 out]
          }
        }
      }
    }
  }
